vi "RegisterForErrors.vi"(8 "error in (no error)":errorcluster, 9 "Observer":refnum<class "Send.lvclass">) -> (0 "error out":errorcluster, 3 "ObserverRegistryCommand_RegisterByLabel out":refnum<class "Observer_RegisterForErrors.lvclass">)   [LabVIEW 2011, in "Messenging.lvlib" / "Observer_RegisterForErrors.lvclass"]
uses:
  Commands/RegisterForErrors/Observer_RegisterForErrors.lvclass
  Interprocess Messenger/Send/Send.lvclass
  Commands/ParentCommand/ObserverRegistryCommand.lvclass
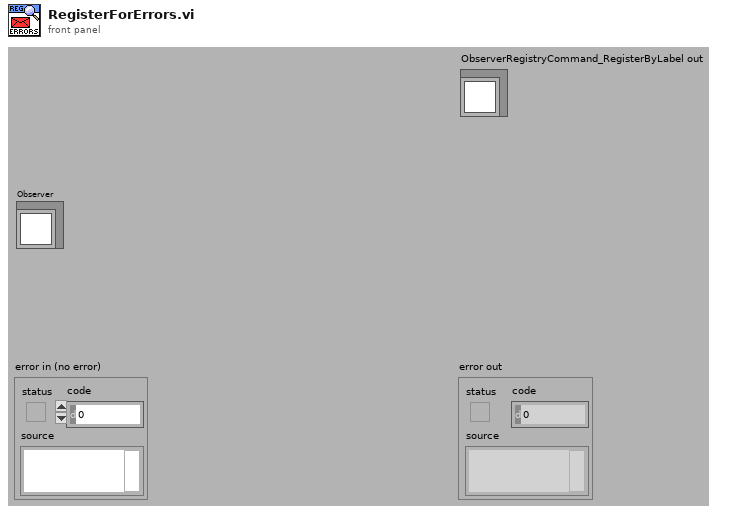
[diagram p1: front panel]
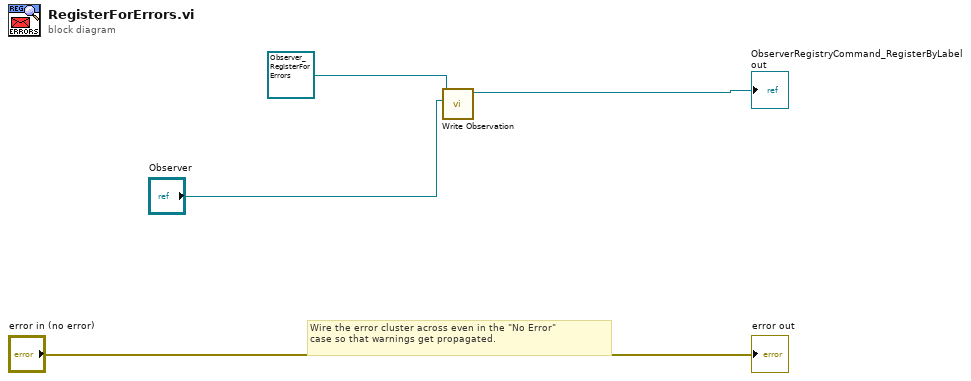
[diagram p0: block diagram]
diagram:
  # "Wire the error cluster across even in the \"No Error\"\ncase so that warnings get propagated."
  n1 = call "Write Observation.vi"("Observer"="Observer", "ObserverRegistryCommand.lvclass in"=refnum<class "Observer_RegisterForErrors.lvclass"> refnum ("ObserverRegistryCommand_RegisterByLabel in")) -> ("ObserverRegistryCommand.lvclass out"=→"ObserverRegistryCommand_RegisterByLabel out":refnum<class "Observer_RegisterForErrors.lvclass">)  [unwired: 1 in, 8 out]
  "error out" <- "error in (no error)"
